vi "DSF.Engine.Interface.Plugin.Write.vi"   [LabVIEW 2016, in "DSF.Engine.lvlib" / "DSF.Engine.Interface.Plugin.lvclass"]
uses:
  DSF.Engine.Interface.Plugin.lvclass
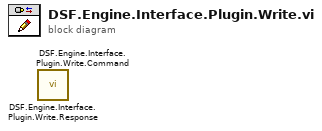
[diagram p0: block diagram]
diagram:
  n1 = call "DSF.Engine.Interface.Plugin.Write.Response.vi"() -> ()  [unwired: 9 in, 3 out]
  n2 = call "DSF.Engine.Interface.Plugin.Write.Command.vi"() -> ()  [unwired: 9 in, 3 out]
